vi "Acquisition_c.vi"() -> (4 "Acquired_Data":dbl(graph))   [LabVIEW 2023]
doc: "This VI acquire data that were generated be the Generator VI.\nTransfer of thet data happens under Queue LV2."
uses:
  Type_Def/Operation_Queue.ctl
panel:
  out "Error_Out":errorcluster
  in  "Error_In":errorcluster
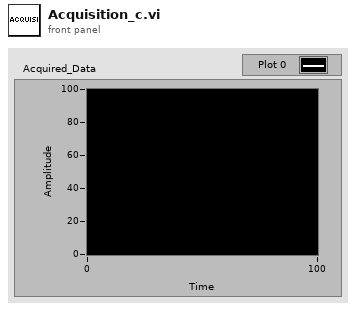
[diagram p1: front panel]
types:
  T1 = typedef "Operation_Queue.ctl" = enum16{"Initialize", "Enqueue", "Dequeue", "Sum"}
  T2 = enum16{"Left Button", "Center Button", "Right Button", "Window Close"}
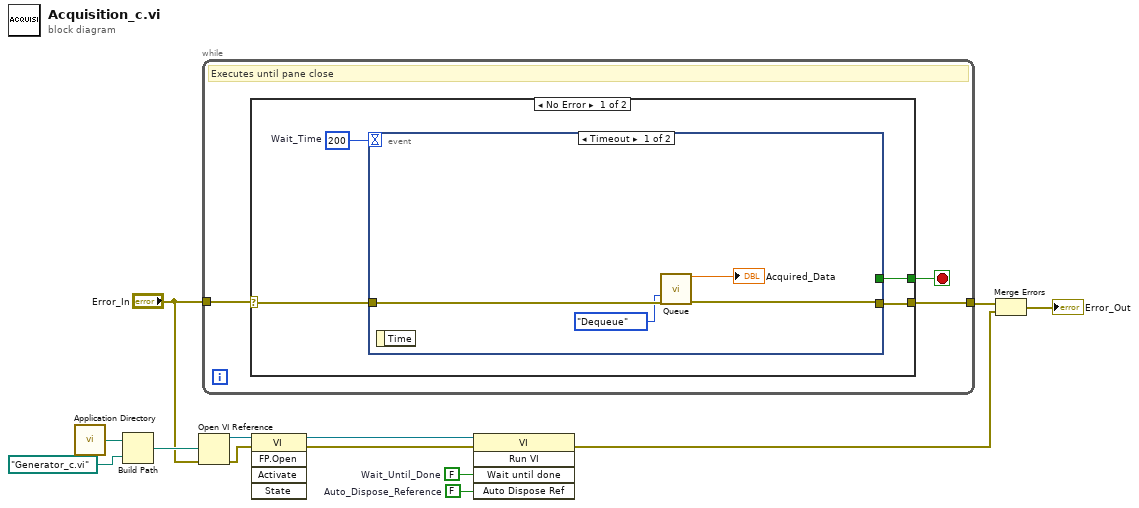
[diagram p0: block diagram]
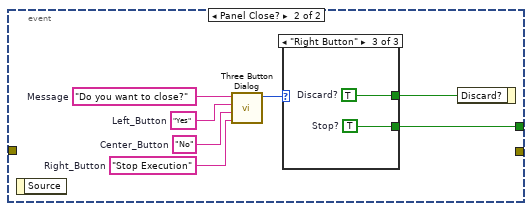
[diagram p2: hidden frame]
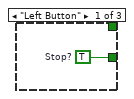
[diagram p3: hidden frame]
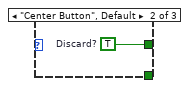
[diagram p4: hidden frame]
diagram:
  w13 = FALSE  # Auto_Dispose_Reference
  w12 = FALSE  # Wait_Until_Done
  n1 = call <vilib>:"Application Directory.vi"() -> ("Application Directory"=w7:path)
  n2 = Build Path(base path=w7, name or relative path=path "Generator_c.vi") -> (appended path=w8:path)
  n3 = Open VI Reference(vi path=w8, error in (no error)="Error_In") -> (vi reference=w10:refnum<vi>, error out=w2:errorcluster)  [unwired: 4 in]
  n4 = while {
    tunnel: "Error_In" -> [w15]
    tunnel: [w14] -> w5
    stop <- w16 stop-if-true
    # "Executes until pane close"
    n5 = case shown="No Error" w15 {
      selector: w15 -> [w18 w36]
      tunnel: [w19 _] -> w16
      tunnel: [w17 w36] -> w14
      frame No Error {
        w20 = 200  # Wait_Time
        n6 = event shown="[0] Timeout" {
          selector: _ -> [_ _]
          dyn-events: _ -> [_ _]
          timeout: w20 -> [_ _]
          tunnel: [_ w25] -> w19
          tunnel: w18 -> [w24 _]
          tunnel: [w23 _] -> w17
          event Timeout {
            n7 = event-data() -> ()  [unwired: 1 in, 1 out]
            n8 = call "Queue.vi"("Operation"=Operation_Queue."Dequeue" ("Operation_Queue"), "Error_In"=w24) -> ("Element_Out"=→"Acquired_Data":dbl, "Error_Out"=w23:errorcluster)  [unwired: 9 in, 3 out]
          }
          event Panel Close? {
            w28 = "Stop Execution"  # Right_Button
            w29 = "No"  # Center_Button
            w30 = "Yes"  # Left_Button
            w31 = "Do you want to close?"  # Message
            n9 = event-data() -> ()  [unwired: 1 in, 1 out]
            n10 = call <vilib>:"Three Button Dialog.vi"("Right Button Text (\"Cancel\")"=w28, "Center Button Text (\"No\")"=w29, "Left Button Text (\"Yes\")"=w30, "message"=w31) -> ("Which Button?"=w27:T2)  [unwired: 7 in]
            n11 = case shown="\"Right Button\"" w27 {
              tunnel: [_ w33 w34] -> w26
              tunnel: [w32 _ w35] -> w25
              frame "Left Button" {
                w32 = TRUE  # Stop?
              }
              frame "Center Button", Default {
                w33 = TRUE  # Discard?
              }
              frame "Right Button" {
                w34 = TRUE  # Discard?
                w35 = TRUE  # Stop?
              }
            }
            n12 = event-data ("Event Filter Node")("Discard?"=w26) -> ()  [unwired: 1 in, 1 out]
          }
        }
      }
      frame Error {
      }
    }
  }
  n13 = invoke on="Invoke Node" class="VI" method="FP.Open"(reference=w10, error in=w2) -> (reference out=w11:refnum<vi>, error out=w6:errorcluster)  [unwired: 3 in, 3 out]
  n14 = invoke on="Invoke Node" class="VI" method="Run VI"(reference=w11, error in=w6, "Wait until done"=w12, "Auto Dispose Ref"=w13) -> (error out=w3:errorcluster)  [unwired: 1 in, 4 out]
  n15 = Merge Errors(w5, w3) -> (→"Error_Out":errorcluster)
